vi "Update Typedef.vi"(8 "error in (no error)":errorcluster, 9 "Data Type":variant, 10 "Name":string, 11 "Application in":refnum<vi>) -> (0 "error out":errorcluster, 1 "Type":variant, 2 "VI Path":path, 3 "Application out":refnum<vi>)   [LabVIEW 2015, in "Scripting.lvlib"]
doc: "Opens the control with the name <B>Name</B> in memory in <B>Application in</B>'s application instance, changes the data type of the control to <B>Data Type</B>, and saves it, supplying the typedef's path at <B>VI Path</B> and type at <B>Type</B>."
uses:
  Scripting.lvlib
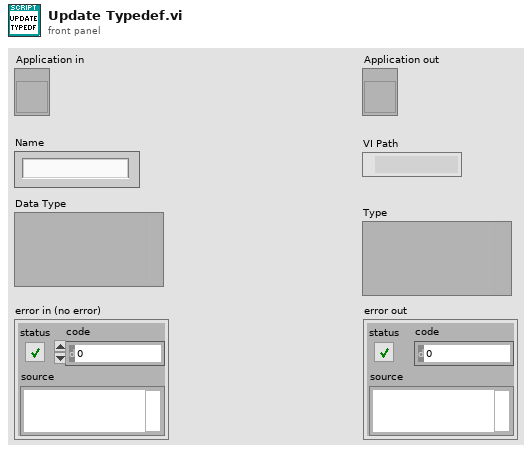
[diagram p1: front panel]
types:
  T1 = enum8{"Probe", "Diagram", "Panel Control", "3D Panel Control", "Dialog Panel Control", "Panel Indicator", "3D Panel Indicator", "Dialog Panel Indicator", "Power PC Control", "Power PC Indicator", "Silver Control", "Silver Indicator"}
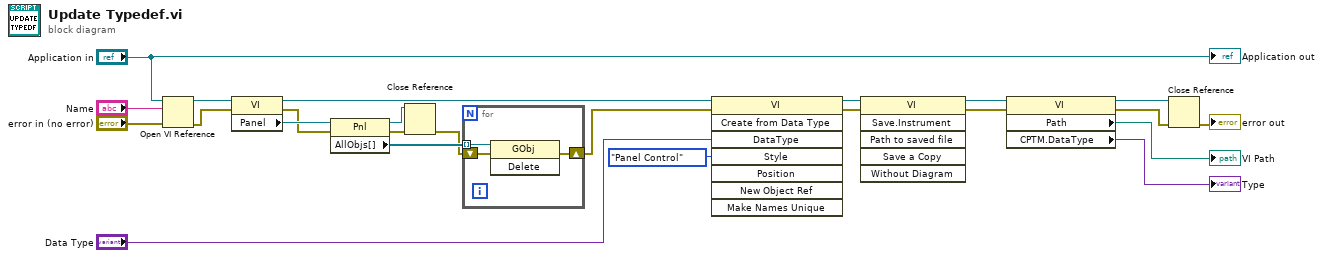
[diagram p0: block diagram]
diagram:
  n1 = Open VI Reference(application reference (local)="Application in", vi path="Name", error in (no error)="error in (no error)") -> (vi reference=w24:refnum<vi>, error out=w23:errorcluster)  [unwired: 3 in]
  n2 = property class="VI"(reference=w24, error in=w23) -> (reference out=w20:refnum<vi>, error out=w19:errorcluster, "Panel"=w22:refnum<vi>)
  n3 = property class="Pnl"(reference=w22, error in=w19) -> (reference out=w1:refnum<vi>, error out=w18:errorcluster, "AllObjs[]"=w21:refnum<vi>[])
  n4 = Close Reference(reference=w1, error in (no error)=w18) -> (error out=w2:errorcluster)
  n5 = for {
    shift-right: [w25] -> w17
    shift-left: w2 -> [w27]
    tunnel: w21 -> [w26] mode=indexing
    n6 = invoke on="Invoke Node" class="GObj" method="Delete"(reference=w26, error in=w27) -> (error out=w25:errorcluster)  [unwired: 1 in, 2 out]
  }
  n7 = invoke class="VI" method="Create from Data Type"(reference=w20, error in=w17, "DataType"="Data Type", "Style"=T1."Panel Control") -> (reference out=w10:refnum<vi>, error out=w13:errorcluster)  [unwired: 4 in, 6 out]
  n8 = invoke class="VI" method="Save.Instrument"(reference=w10, error in=w13) -> (reference out=w6:refnum<vi>, error out=w8:errorcluster)  [unwired: 4 in, 4 out]
  n9 = property class="VI"(reference=w6, error in=w8) -> (reference out=w5:refnum<vi>, error out=w7:errorcluster, "Path"=→"VI Path":path, "CPTM.DataType"=→"Type":variant)
  n10 = Close Reference(reference=w5, error in (no error)=w7) -> (error out=→"error out":errorcluster)
  "Application out" <- "Application in"
